vi "AUTO DRIVE SYS.vi"() -> ()   [LabVIEW 2023]
uses:
  Global odometry.vi
  <vilib>/Rock Robotics/WPI/ThirdParty/JAS_Junk/TrajLib/Trajectory_Library.lvlib
  Global INIT.vi
  <vilib>/Rock Robotics/WPI/ThirdParty/JAS_Junk/TrajLib/TypeDef/TIMER.ctl
panel:
  in  "rotation target":dbl
  out "wheel\nrotations":dbl[](array[numeric])
  out "throttle delta":dbl
  out "-1, 0, 1":dbl
  out "Heading\nchange":dbl
  in  "Throttle\nincrease":dbl format="%#_13g"
  out "Throttle":dbl format="%#_13g"
  out "Heading\ncurrent":dbl
  out "Heading\ninitial":dbl
  out "error out":errorcluster
  in  "error in":errorcluster
  out "elapsed seconds":dbl
  out "Timer\nSTART":T1 {"Accumulated TIme" format="%13.5p"; "StartTime" format="%13.5p"}
  out "out Timer":T1 {"Accumulated TIme" format="%13.5p"; "StartTime" format="%13.5p"}
  in  "DRIVE BRNG (deg)":u32
  in  "DRIVE\nlimit (ms)":u32
  in  "DRIVE OUT\nVBus":dbl
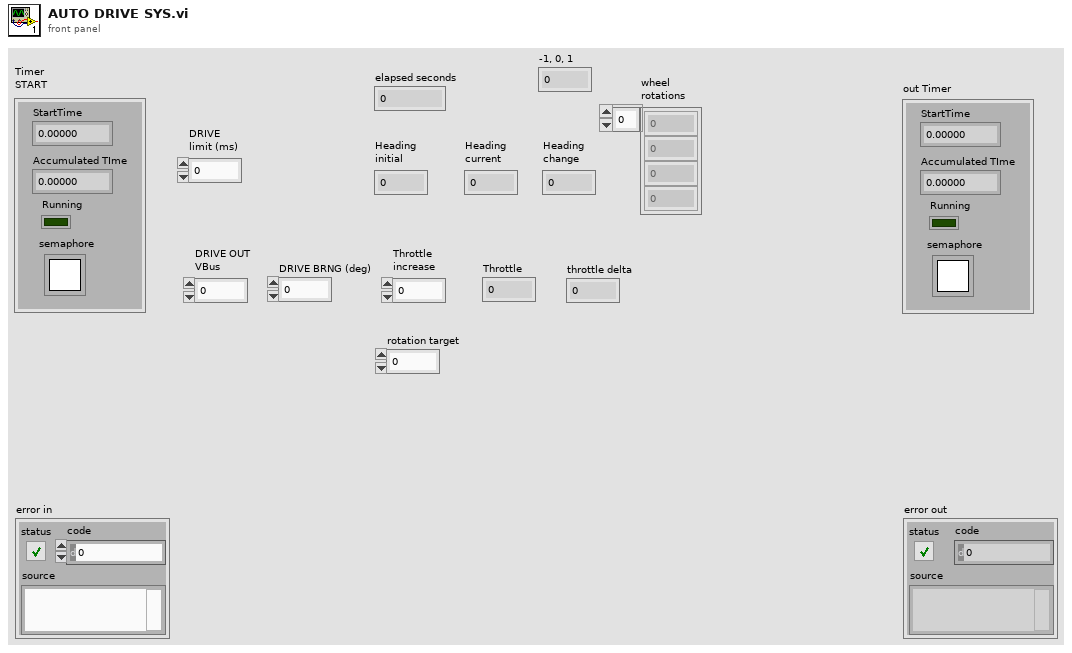
[diagram p1: front panel]
types:
  T1 = typedef "Trajectory_Library.lvlib/TIMER.ctl" = cluster{"StartTime":dbl, "Accumulated TIme":dbl, "Running":bool, "semaphore":T2}
  T2 = typedef "Semaphore RefNum" = refnum<k1>
  T3 = typedef "ctrl swerve motor.ctl" = cluster{"description":string, "MOTOR SELECT":T4, "Installed?":bool, "CAN ID":u8, "refnum name":string, "Invert":bool, "Idle Mode":T5, "Current limiting":T6, "MOTOR PIDF coefficients":T7, "gear ratio":dbl}
  T4 = typedef "ctrl MOTOR SELECT.ctl" = i16
  T5 = typedef "Spark MAX Idle Mode.ctl" = enum16{"Coast", "Brake"}
  T6 = typedef "ctrl Spark MAX current limiting.ctl" = cluster{"Linearized":bool, "Free Speed (A)":dbl, "Primay (A)":dbl, "Limit RPM (0)":u32}
  T7 = typedef "ctrl motor PIDF coefficients.ctl" = cluster{"PIDF":cluster{"P Gain":dbl, "I Gain":dbl, "D Gain":dbl, "F Gain":dbl, "I Zone":dbl, "Min Output":dbl, "Max Output":dbl}, "Smart Motion":T8}
  T8 = typedef "Spark MAX Smart Motion Parameters.ctl" = cluster{"Max Velocity":dbl, "Max Acceleration":dbl, "Minimum Velocity Output":dbl, "Allowed Closed Loop Error":dbl}
  T9 = typedef "WPI_MotorControlDeviceRef.ctl" = cluster{"DeviceStatus":errorcluster, "Type":T10, "PWM":cluster{"PWM Channel":T11, "DeadBand":T12}, "CAN":cluster{"Device Number":u8, "SetOutput VI Ref":variant, "GetOutput VI Ref":variant, "Enable VI Ref":variant, "Disable VI Ref":variant, "Data":variant}, "Invert":bool, "DIO PWM":cluster{"PWM \"Enable\" Channel":T11, "DIOChannel":T13, "PWM Rate":dbl}}
  T10 = typedef "WPI_MotorControlType.ctl" = enum16{"PWM", "CAN", "DIO PWM"}
  T11 = typedef "FPGA_DIOPWMChannel.ctl" = enum8{"PWM 0", "PWM 1", "PWM 2", "PWM 3", "PWM 4", "PWM 5", "PWM 6", "PWM 7", "PWM 8", "PWM 9", "PWM MXP 0", "PWM MXP 1", "PWM MXP 2", "PWM MXP 3", "PWM MXP 4", "PWM MXP 5", "PWM MXP 6", "PWM MXP 7", "PWM MXP 8", "PWM MXP 9", "Invalid"}
  T12 = typedef "WPI_PWMDeadband.ctl" = cluster{"Name":string, "maxPositivePwm":i32, "minPositivePwm":i32, "centerPwm":i32, "maxNegativePwm":i32, "minNegativePwm":i32, "angularRange":u16}
  T13 = typedef "FPGA_DIOChannel.ctl" = enum8{"DIO 0", "DIO 1", "DIO 2", "DIO 3", "DIO 4", "DIO 5", "DIO 6", "DIO 7", "DIO 8", "DIO 9", "DIO MXP 0", "DIO MXP 1", "DIO MXP 2", "DIO MXP 3", "DIO MXP 4", "DIO MXP 5", "DIO MXP 6", "DIO MXP 7", "DIO MXP 8", "DIO MXP 9", "DIO MXP 10", "DIO MXP 11", "DIO MXP 12", "DIO MXP 13", "DIO MXP 14", "DIO MXP 15", "SPI Port CS1", "SPI Port CS2", "SPI Port CS3", "SPI Port MISO", "SPI Port MOSI", "Invalid"}
  T14 = cluster{"Yaw":dbl, "Roll":dbl, "Pitch":dbl, "Heading":dbl, "Fused Heading":dbl}
  T15 = typedef "ctrl driver input.ctl" = cluster{"Jx":dbl, "Jy":dbl, "Jr ":dbl, "R":dbl, "theta (deg)":dbl, "theta (rad)":dbl, "PARK":bool}
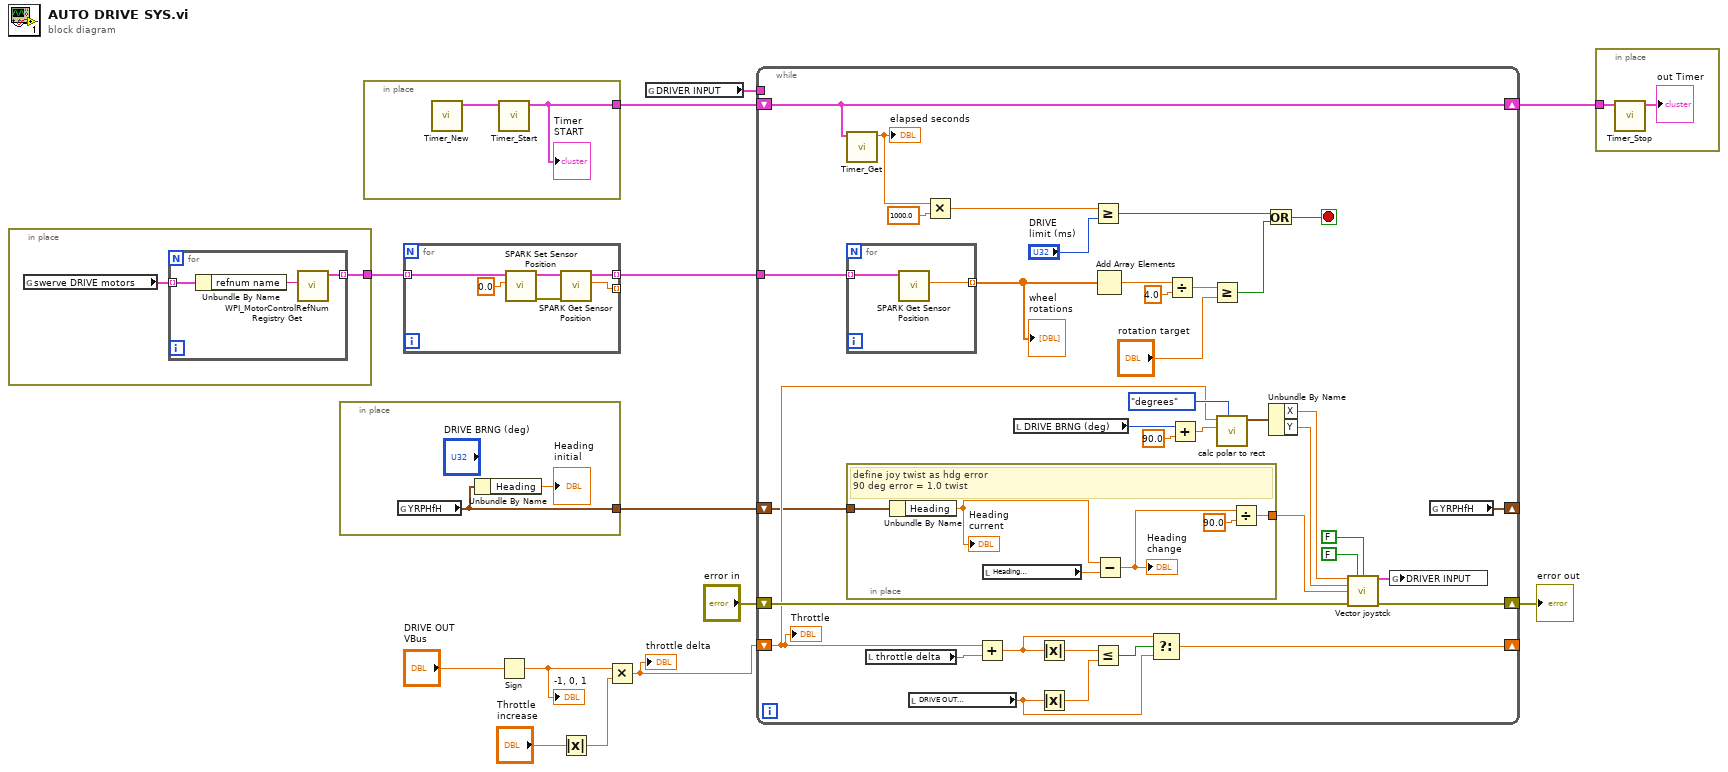
[diagram p0: block diagram]
diagram:
  n1 = in-place {
    in-place-border: [w14] -> w2
    n2 = global read "Global INIT.vi" "swerve DRIVE motors"() -> (w15:T3[])
    n3 = for {
      tunnel: w15 -> [w18] mode=indexing
      tunnel: [w16] -> w14 mode=indexing
      n4 = Unbundle By Name(w18) -> ("refnum name"=w17:string)
      n5 = call <vilib>:"WPI_MotorControlRefNum Registry Get.vi"("refnum name"=w17) -> ("MotorControlDevRef"=w16:T9)  [unwired: 9 in, 1 out]
    }
  }
  n6 = in-place {
    in-place-border: [w20] -> w8
    n7 = global read "Global odometry.vi" "YRPHfH"() -> (w20:T14)
    n8 = Unbundle By Name(w20) -> ("Heading"=→"Heading\ninitial":dbl)
  }
  n9 = in-place {
    in-place-border: [w21] -> w13
    n10 = call <vilib>:"Timer_New.vi"() -> ("TIMER"=w22:T1)  [unwired: 11 in]
    n11 = call <vilib>:"Timer_Start.vi"("in Timer"=w22) -> ("out Timer"=w21:T1)  [unwired: 10 in]
    "Timer\nSTART" <- w21
  }
  n12 = for {
    tunnel: w2 -> [w28] mode=indexing
    tunnel: [w24] -> w1 mode=indexing
    tunnel: [w23] -> _ mode=indexing
    n13 = call <vilib>:"SPARK Set Sensor Position.vi"("Position"=0.0, "MotorControlDeviceRef"=w28) -> ("error out"=w26:errorcluster, "MotorControlDeviceRef"=w25:T9)  [unwired: 8 in]
    n14 = call <vilib>:"SPARK Get Sensor Position.vi"("error in (no error)"=w26, "MotorControlDevRef in"=w25) -> ("Sensor Position"=w23:dbl, "MotorControlDevRef out"=w24:T9)  [unwired: 6 in, 2 out]
  }
  n15 = Sign(1:"DRIVE OUT\nVBus") -> (0:w3:dbl)
  "-1, 0, 1" <- w3
  n16 = Absolute Value(x="Throttle\nincrease") -> (abs(x)=w6:dbl)
  n17 = Multiply(x=w3, y=w6) -> (x*y=w4:dbl)
  "throttle delta" <- w4
  n18 = global read "Global odometry.vi" "DRIVER INPUT"() -> (w11:T15)
  n19 = while {
    tunnel: w11 -> [_]
    shift-right: [w62] -> w9
    shift-left: "error in" -> [w63]
    shift-right: [w51] -> w12
    shift-left: w13 -> [w51]
    shift-right: [w48] -> _
    shift-left: w8 -> [w38]
    shift-right: [w45] -> _
    shift-left: w4 -> [w47]
    tunnel: w1 -> [w36]
    stop <- w33 stop-if-true
    n20 = call <vilib>:"Timer_Get.vi"("TIMER"=w51) -> ("CurrentTImer"=w53:dbl)  [unwired: 10 in]
    "elapsed seconds" <- w53
    n21 = for {
      tunnel: w36 -> [w73] mode=indexing
      tunnel: [w72] -> w32 mode=indexing
      n22 = call <vilib>:"SPARK Get Sensor Position.vi"("MotorControlDevRef in"=w73) -> ("Sensor Position"=w72:dbl)  [unwired: 7 in, 3 out]
    }
    "wheel\nrotations" <- w32
    n23 = in-place {
      in-place-border: w38 -> [w69]
      in-place-border: [w66] -> w37
      # "define joy twist as hdg error\n90 deg error = 1.0 twist"
      n24 = Unbundle By Name(w69) -> ("Heading"=w71:dbl)
      "Heading\ncurrent" <- w71
      n25 = local read "Heading\ninitial"() -> (w70:dbl)
      n26 = Subtract(x=w71, y=w70) -> (x-y=w68:dbl)
      "Heading\nchange" <- w68
      n27 = Divide(x=w68, y=90.0) -> (x/y=w66:dbl)
    }
    n28 = local read "throttle delta"() -> (w46:dbl)
    n29 = local read "DRIVE OUT\nVBus"() -> (w40:dbl)
    n30 = Multiply(x=w53, y=1000.0) -> (x*y=w54:dbl)
    n31 = Add(x=w47, y=w46) -> (x+y=w41:dbl)
    n32 = local read "DRIVE BRNG (deg)"() -> (w59:u32)
    n33 = Absolute Value(x=w41) -> (abs(x)=w44:dbl)
    n34 = Absolute Value(x=w40) -> (abs(x)=w43:dbl)
    n35 = Greater Or Equal?(x=w54, y="DRIVE\nlimit (ms)") -> (x >= y?=w50:bool)
    n36 = Less Or Equal?(x=w44, y=w43) -> (x <= y?=w42:bool)
    n37 = Add Array Elements(numeric array=w32) -> (sum=w35:dbl)
    n38 = Select(t=w41, s=w42, f=w40) -> (s? t:f=w45:dbl)
    n39 = Divide(x=w35, y=4.0) -> (x/y=w31:dbl)
    n40 = Add(x=w59, y=90.0) -> (x+y=w60:dbl)
    n41 = Greater Or Equal?(x=w31, y="rotation target") -> (x >= y?=w29:bool)
    n42 = call "calc polar to rect.vi"("units"=enum16{"degrees", "radians"}."degrees", "angle"=w60, "mag"=w47) -> ("XY"=w61:cluster{"X":dbl, "Y":dbl})  [unwired: 8 in]
    n43 = Or(x=w50, y=w29) -> (x .or. y?=w33:bool)
    n44 = Unbundle By Name(w61) -> ("X"=w56:dbl, "Y"=w55:dbl)
    n45 = call "Vector joystck.vi"("Jx input"=w56, "apply\nFILTER"=FALSE ("apply\nFILTER"), "Reset\nFILTER"=FALSE ("Reset\nFILTER"), "Jy input"=w55, "Jr input"=w37, "error in (no error)"=w63) -> ("output cluster"=w49:T15, "error out"=w62:errorcluster)  [unwired: 8 in]
    n46 = global write "Global odometry.vi" "DRIVER INPUT"(w49) -> ()
    n47 = global read "Global odometry.vi" "YRPHfH"() -> (w48:T14)
    "Throttle" <- w47
  }
  "error out" <- w9
  n48 = in-place {
    in-place-border: w12 -> [w75]
    n49 = call <vilib>:"Timer_Stop.vi"("in Timer"=w75) -> ("out Timer"=→"out Timer":T1)  [unwired: 10 in]
  }
